vi "CC Edit FITS Header.vi"() -> ()   [LabVIEW 2024]
uses:
  Detector/FITS/FITS enum Data Type.ctl
  Detector/FITS/FITS cluster Header Row.ctl
panel:
  in  "Close":bool
  in  "Units":string
  in  "Save Header":bool
  in  "Add/Replace":bool
  in  "Comment":string
  in  "Value":string
  in  "Header Field":string(combo)
  in  "FITS Header":i32(listbox)
  in  "Type":T1
  # "These FITS header fields will be added to all images"
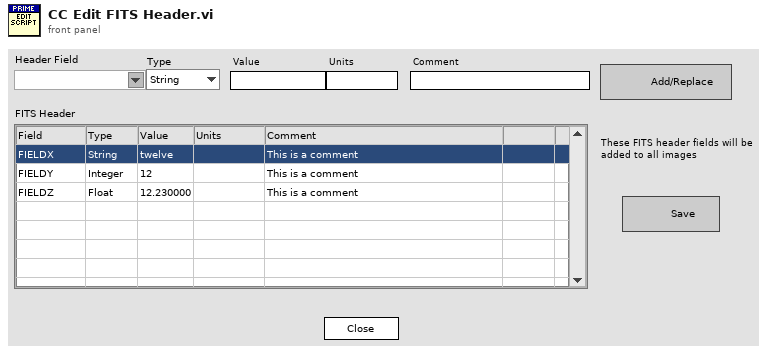
[diagram p1: front panel]
types:
  T1 = typedef "FITS enum Data Type.ctl" = enum16{"String", "Integer", "Float"}
  T2 = typedef "FITS cluster Header Row.ctl" = cluster{"Field Name":string, "Type":T1, "Value":string, "Comment":string, "Units":string}
  T3 = cluster{"state":refnum<user-event>, "Hdr Map":map{string, T2}}
  T4 = typedef "RIMAS Detector Config.ctl" = cluster{"Detector":u16, "Offsets":u16[][], "Detector Computer":T5, "FITS hdr template0":path, "FITS hdr template1":path, "FITS Data File Path":path, "FITS Detector Settings":T6, "Sim Folder":path, "Integration Mode":T7, "Integration Time":dbl, "Frame Int Time":dbl}
  T5 = typedef "RIMAS Detector Server Config.ctl" = cluster{"Machine":string, "Password":string, "FITS File Path":string, "Port":u16, "Header Path":string, "Name":string}
  T6 = typedef "RIMAS Observation Config.ctl" = cluster{"Exp Time Short":dbl, "# of Frames":dbl, "Exp Time Long":dbl, "# of Groups":dbl, "Object Name":string, "Object":string, "Obs Type":string, "Image Type":string, "Observer":string, "Observer Affiliation":string}
  T7 = typedef "Detector enum Detector Integration Mode.ctl" = enum16{"SSR", "CDS", "MEAN", "MEDIAN", "MODE", "MIIN", "MAX"}
  T8 = typedef "LVPoint32TypeDef.ctl" = cluster{"Horizontal":i32, "Vertical":i32}
  T9 = typedef "LVRowAndColumnTypeDef.ctl" = cluster{"Row":i32, "Column":i32}
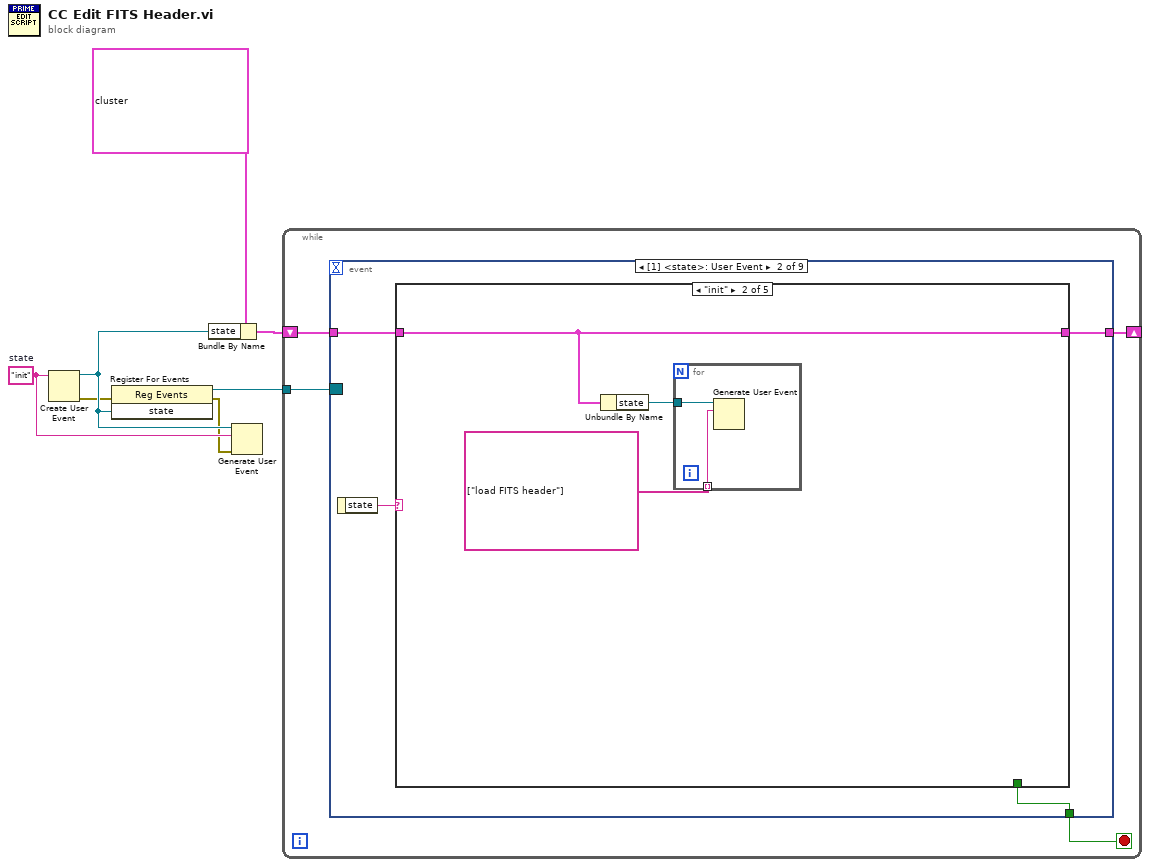
[diagram p0: block diagram]
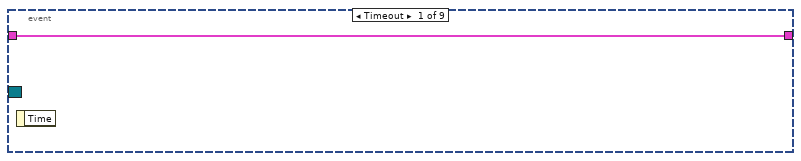
[diagram p2: hidden frame]
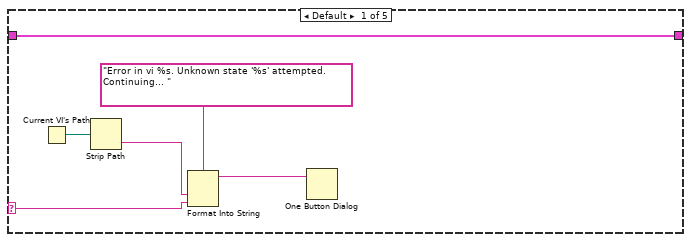
[diagram p3: hidden frame]
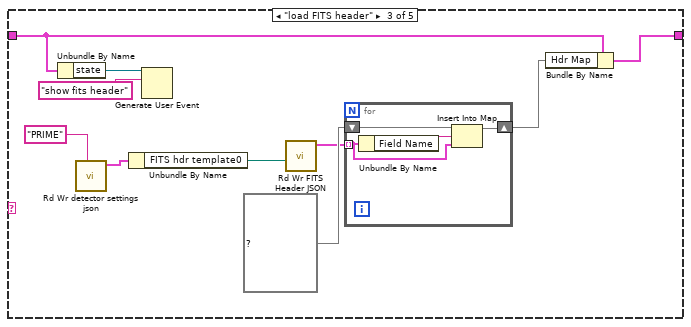
[diagram p4: hidden frame]
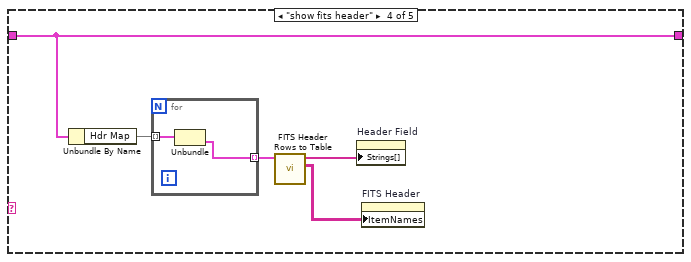
[diagram p5: hidden frame]
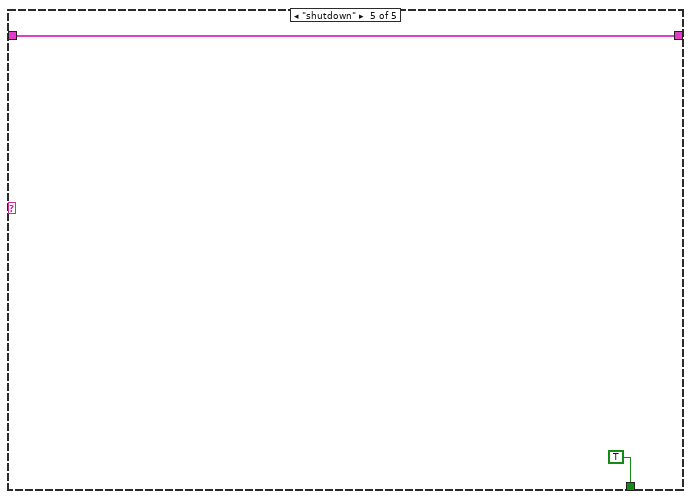
[diagram p6: hidden frame]
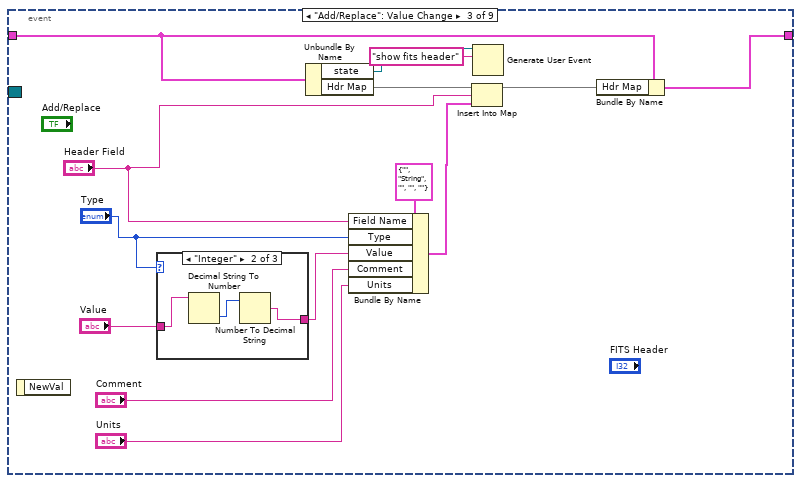
[diagram p7: hidden frame]
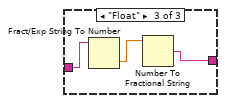
[diagram p9: hidden frame]
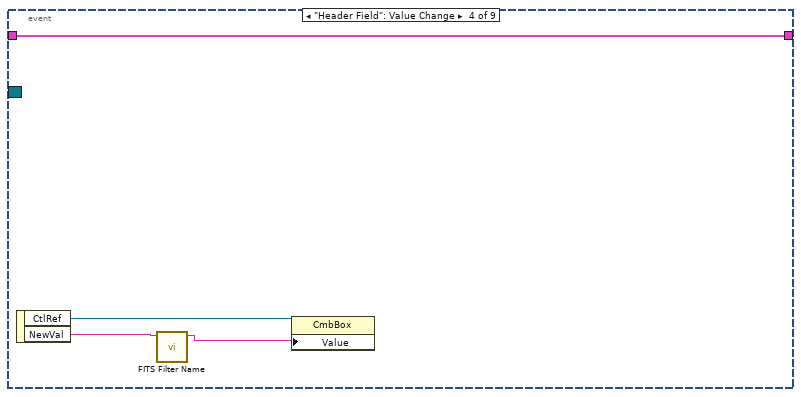
[diagram p10: hidden frame]
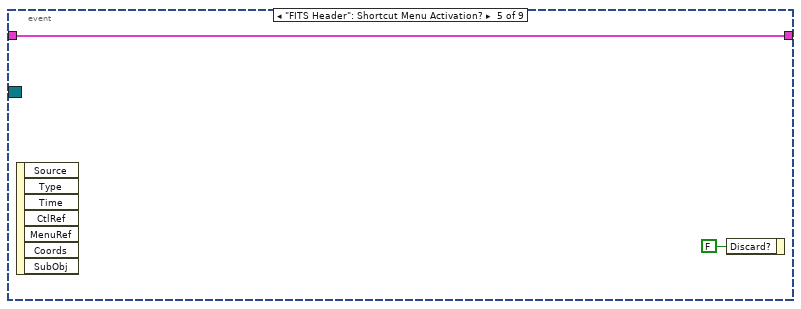
[diagram p11: hidden frame]
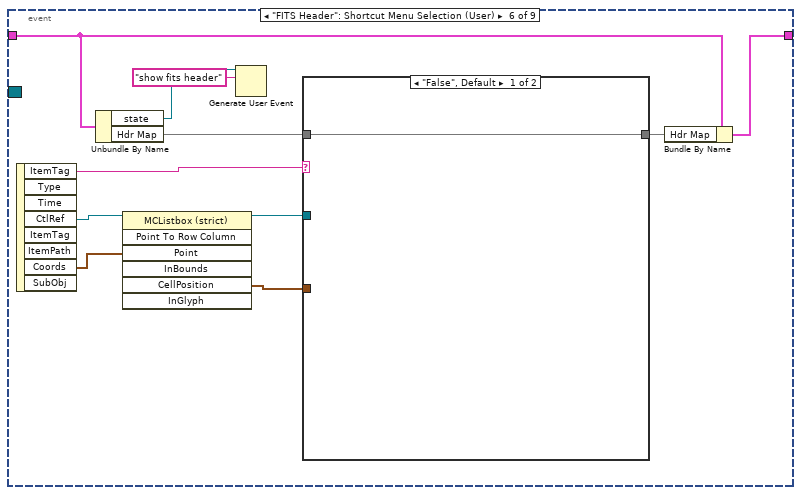
[diagram p12: hidden frame]
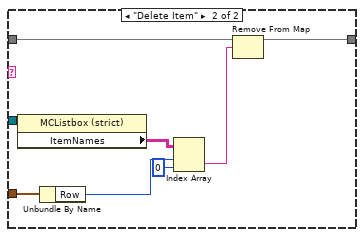
[diagram p13: hidden frame]
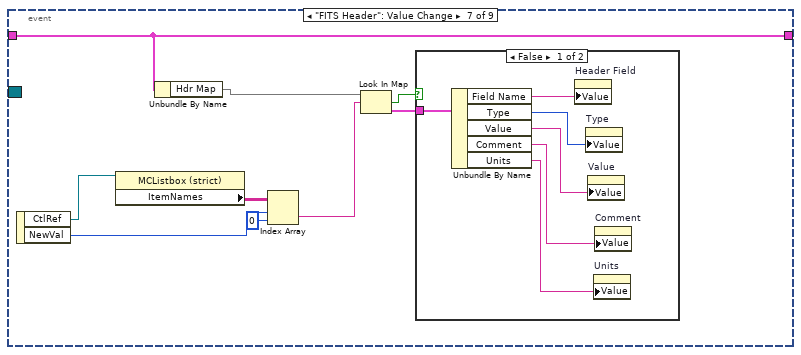
[diagram p14: hidden frame]
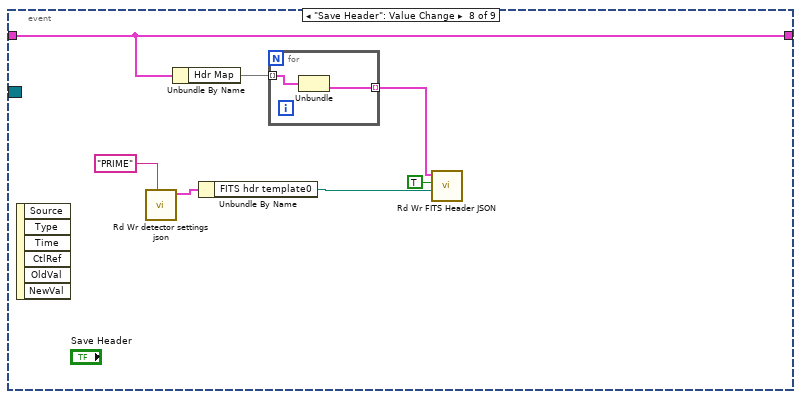
[diagram p16: hidden frame]
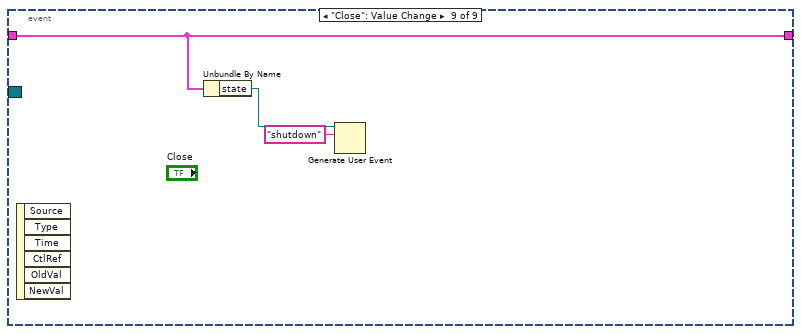
[diagram p17: hidden frame]
diagram:
  w3 = "init"  # state
  n1 = Create User Event(user event datatype=w3) -> (user event=w5:refnum<user-event>, error out=w1:errorcluster)  [unwired: 1 in]
  n2 = register-events(error in=w1, w5) -> (reference out=w4:refnum<event-registration>, error out=w2:errorcluster)  [unwired: 1 in]
  n3 = Bundle By Name(cluster=T3 {"state"=refnum, "Hdr Map"={}}, "state"=w5) -> (w6:T3)
  n4 = Generate User Event(user event=w5, event data cluster=w3, error in=w2) -> ()  [unwired: 1 in, 2 out]
  n5 = while {
    tunnel: w4 -> [w11]
    shift-right: [w9] -> _
    shift-left: w6 -> [w10]
    stop <- w8 stop-if-true
    n6 = event shown="[1] <state>: User Event" {
      selector: w11 -> [_ _ _ _ _ _ _ _ _]
      dyn-events: _ -> [_ _ _ _ _ _ _ _ _]
      timeout: _ -> [_ _ _ _ _ _ _ _ _]
      tunnel: w10 -> [w12 w15 w63 w75 w77 w80 w102 w116 w124]
      tunnel: [w12 w14 w64 w75 w77 w81 w102 w116 w124] -> w9
      tunnel: [_ w13 _ _ _ _ _ _ _] -> w8
      event Timeout {
        n7 = event-data() -> ()  [unwired: 1 in, 1 out]
      }
      event User Event {
        n8 = event-data() -> ("state"=w16:string)  [unwired: 1 in]
        n9 = case shown="\"init\"" w16 {
          selector: w16 -> [w21 _ _ _ _]
          tunnel: w15 -> [w17 w23 w30 w44 w50]
          tunnel: [w17 w23 w35 w44 w50] -> w14
          tunnel: [_ _ _ _ TRUE] -> w13
          frame Default {
            n10 = Current VI's Path() -> (path=w20:path)
            n11 = Strip Path(path=w20) -> (name=w19:string)  [unwired: 1 out]
            n12 = Format Into String(format string="Error in vi %s. Unknown state '%s' attempted. Continuing... ", w19, w21) -> (resulting string=w18:string)  [unwired: 2 in, 1 out]
            n13 = One Button Dialog(message=w18) -> ()  [unwired: 1 in, 1 out]
          }
          frame "init" {
            n14 = Unbundle By Name(w23) -> ("state"=w25:refnum<user-event>)
            n15 = for {
              tunnel: w25 -> [w27]
              tunnel: string[] ["load FITS header"] -> [w26] mode=indexing
              n16 = Generate User Event(user event=w27, event data cluster=w26) -> ()  [unwired: 2 in, 2 out]
            }
          }
          frame "load FITS header" {
            n17 = Unbundle By Name(w30) -> ("state"=w29:refnum<user-event>)
            n18 = call "Rd Wr detector settings json.vi"("Detector Name"="PRIME") -> ("Detector Config"=w36:T4)  [unwired: 9 in, 1 out]
            n19 = Unbundle By Name(w36) -> ("FITS hdr template0"=w34:path)
            n20 = Generate User Event(user event=w29, event data cluster="show fits header" ("event data")) -> ()  [unwired: 2 in, 2 out]
            n21 = call "Rd Wr FITS Header JSON.vi"("FITS Template"=w34) -> ("FITS Hdr Rows"=w31:T2[])  [unwired: 9 in, 1 out]
            n22 = for {
              tunnel: w31 -> [w39] mode=indexing
              shift-right: [w38] -> w32
              shift-left: map{string, T2} {} ("Hdr Map") -> [w41]
              n23 = Unbundle By Name(w39) -> ("Field Name"=w40:string)
              n24 = Insert Into Map(map in=w41, key=w40, value=w39) -> (map out=w38:map{string, T2})  [unwired: 2 out]
            }
            n25 = Bundle By Name(cluster=w30, "Hdr Map"=w32) -> (w35:T3)
          }
          frame "show fits header" {
            n26 = Unbundle By Name(w44) -> ("Hdr Map"=w43:map{string, T2})
            n27 = for {
              tunnel: w43 -> [w48] mode=indexing
              tunnel: [w47] -> w42 mode=indexing
              n28 = Unbundle(w48) -> (w47:T2)  [unwired: 1 out]
            }
            n29 = call "FITS Header Rows to Table.vi"("FITS Hdr Rows"=w42) -> ("table"=w45:string[][], "Keywords"=w46:string[])  [unwired: 9 in]
            n30 = property on="Header Field" class="CmbBox"("Strings[]"=w46) -> ()  [unwired: 2 in, 2 out]
            n31 = property on="FITS Header" class="MCListbox (strict)"("ItemNames"=w45) -> ()  [unwired: 2 in, 2 out]
          }
          frame "shutdown" {
          }
        }
      }
      event "Add/Replace": Value Change {
        n32 = event-data() -> ()  [unwired: 1 in, 1 out]
        n33 = case shown="\"Integer\"" "Type" {
          tunnel: "Value" -> [w65 w68 w71]
          tunnel: [w65 w66 w69] -> w52
          frame "String", Default {
          }
          frame "Integer" {
            n34 = Decimal String To Number(string=w68) -> (number=w67:i32)  [unwired: 2 in, 1 out]
            n35 = Number To Decimal String(number=w67) -> (decimal integer string=w66:string)  [unwired: 1 in]
          }
          frame "Float" {
            n36 = Fract/Exp String To Number(string=w71) -> (number=w70:dbl)  [unwired: 3 in, 1 out]
            n37 = Number To Fractional String(number=w70) -> (F-format string=w69:string)  [unwired: 3 in]
          }
        }
        n38 = Unbundle By Name(w63) -> ("state"=w56:refnum<user-event>, "Hdr Map"=w59:map{string, T2})
        n39 = Bundle By Name(cluster=T2 {"Field Name"="", "Type"=enum."String", "Value"="", "Comment"="", "Units"=""} ("FITS Hdr Row"), "Field Name"="Header Field", "Type"="Type", "Value"=w52, "Comment"="Comment", "Units"="Units") -> (w58:T2)
        n40 = Insert Into Map(map in=w59, key="Header Field", value=w58) -> (map out=w57:map{string, T2})  [unwired: 2 out]
        n41 = Generate User Event(user event=w56, event data cluster="show fits header" ("event data")) -> ()  [unwired: 2 in, 2 out]
        n42 = Bundle By Name(cluster=w63, "Hdr Map"=w57) -> (w64:T3)
      }
      event "Header Field": Value Change {
        n43 = event-data() -> ("CtlRef"=w74:refnum<vi>, "NewVal"=w73:string)  [unwired: 1 in]
        n44 = call "FITS Filter Name.vi"("Hdr Name"=w73) -> ("Filtered Name"=w72:string)  [unwired: 9 in, 1 out]
        n45 = property class="CmbBox"(reference=w74, "Value"=w72) -> ()  [unwired: 1 in, 2 out]
      }
      event "FITS Header": Shortcut Menu Activation? {
        n46 = event-data() -> ()  [unwired: 1 in, 7 out]
        n47 = event-data("Discard?"=FALSE) -> ()  [unwired: 1 in, 1 out]
      }
      event "FITS Header": Shortcut Menu Selection (User) {
        n48 = event-data() -> ("ItemTag"=w86:string, "CtlRef"=w88:refnum<vi>, "Coords"=w87:T8)  [unwired: 1 in, 5 out]
        n49 = Unbundle By Name(w80) -> ("state"=w79:refnum<user-event>, "Hdr Map"=w83:map{string, T2})
        n50 = invoke class="MCListbox (strict)" method="Point To Row Column"(reference=w88, "Point"=w87) -> (reference out=w84:refnum<vi>, "CellPosition"=w85:T9)  [unwired: 5 in, 5 out]
        n51 = Generate User Event(user event=w79, event data cluster="show fits header" ("event data")) -> ()  [unwired: 2 in, 2 out]
        n52 = case shown="\"False\", Default" w86 {
          tunnel: w85 -> [_ w97]
          tunnel: w84 -> [_ w96]
          tunnel: w83 -> [w89 w92]
          tunnel: [w89 w90] -> w82
          frame "False", Default {
          }
          frame "Delete Item" {
            n53 = property class="MCListbox (strict)"(reference=w96) -> ("ItemNames"=w95:string[][])  [unwired: 1 in, 2 out]
            n54 = Unbundle By Name(w97) -> ("Row"=w94:i32)
            n55 = Index Array(array=w95, index (row)=w94, index (col)=0 ("disabled index (col)")) -> (element=w91:string)
            n56 = Remove From Map(10:w91, 11:w92) -> (3:w90:map{string, T2})  [unwired: 2 out]
          }
        }
        n57 = Bundle By Name(cluster=w80, "Hdr Map"=w82) -> (w81:T3)
      }
      event "FITS Header": Value Change {
        n58 = event-data() -> ("CtlRef"=w106:refnum<vi>, "NewVal"=w104:i32)  [unwired: 1 in]
        n59 = property class="MCListbox (strict)"(reference=w106) -> ("ItemNames"=w105:string[][])  [unwired: 1 in, 2 out]
        n60 = Unbundle By Name(w102) -> ("Hdr Map"=w101:map{string, T2})
        n61 = Index Array(array=w105, index (row)=w104, index (col)=0 ("disabled index (col)")) -> (element=w100:string)
        n62 = Look In Map(map=w101, key=w100) -> (key not found?=w99:bool, value=w98:T2)  [unwired: 1 in]
        n63 = case shown="False" w99 {
          tunnel: w98 -> [w112 _]
          frame False {
            n64 = Unbundle By Name(w112) -> ("Field Name"=w111:string, "Type"=w110:T1, "Value"=w109:string, "Comment"=w108:string, "Units"=w107:string)
            n65 = property on="Header Field" class="CmbBox"("Value"=w111) -> ()  [unwired: 2 in, 2 out]
            n66 = property on="Type" class="Enum (strict)"("Value"=w110) -> ()  [unwired: 2 in, 2 out]
            n67 = property on="Value" class="Str"("Value"=w109) -> ()  [unwired: 2 in, 2 out]
            n68 = property on="Units" class="Str"("Value"=w107) -> ()  [unwired: 2 in, 2 out]
            n69 = property on="Comment" class="Str"("Value"=w108) -> ()  [unwired: 2 in, 2 out]
          }
          frame True {
          }
        }
      }
      event "Save Header": Value Change {
        n70 = event-data() -> ()  [unwired: 1 in, 6 out]
        n71 = call "Rd Wr detector settings json.vi"("Detector Name"="PRIME") -> ("Detector Config"=w118:T4)  [unwired: 9 in, 1 out]
        n72 = Unbundle By Name(w116) -> ("Hdr Map"=w115:map{string, T2})
        n73 = Unbundle By Name(w118) -> ("FITS hdr template0"=w117:path)
        n74 = for {
          tunnel: w115 -> [w121] mode=indexing
          tunnel: [w120] -> w114 mode=indexing
          n75 = Unbundle(w121) -> (w120:T2)  [unwired: 1 out]
        }
        n76 = call "Rd Wr FITS Header JSON.vi"("FITS Template"=w117, "Write? (F:Read)"=TRUE, "FITS Hdr Rows"=w114) -> ()  [unwired: 7 in, 2 out]
      }
      event "Close": Value Change {
        n77 = event-data() -> ()  [unwired: 1 in, 6 out]
        n78 = Unbundle By Name(w124) -> ("state"=w123:refnum<user-event>)
        n79 = Generate User Event(user event=w123, event data cluster="shutdown" ("event data")) -> ()  [unwired: 2 in, 2 out]
      }
    }
  }
